vi "createDestinationDirectory.vi"(8 "error in (no error)":errorcluster, 11 "PolymorphicStructure in":refnum<class "PolymorphicStructure.lvclass">) -> (0 "error out":errorcluster, 2 "instanceDirectories":path[](array[path]), 3 "PolymorphicStructure out":refnum<class "PolymorphicStructure.lvclass">)   [LabVIEW 2012, in "PolymorphicStructure.lvclass"]
uses:
  PolymorphicStructure.lvclass
  PolymorphicStructure.lvclass/PolymorphicStructure.ctl
  <vilib>/LabVIEW Icon API/API_Text.ctl
  Directory/Directory.lvclass
  <vilib>/LabVIEW Icon API/LabVIEW Icon API.lvlib
  VirtualInstrument/VirtualInstrument.lvclass
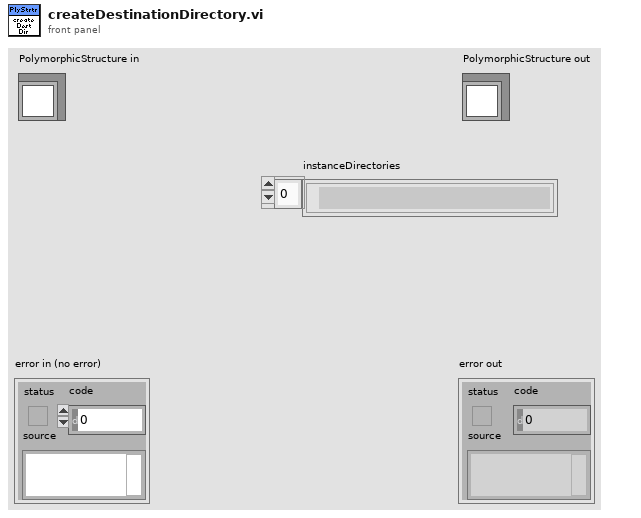
[diagram p1: front panel]
types:
  T1 = typedef "LabVIEW Icon API.lvlib/API_Text.ctl" = cluster{"Line 1 text":string, "Line 2 text":string, "Line 3 text":string, "Line 4 text":string}
  T2 = enum32{"invalid VI type", "Standard VI", "Control VI", "Global VI", "Polymorphic VI", "Configuration VI", "SubSystem", "Facade VI", "Method VI", "Statechart Diagram VI"}
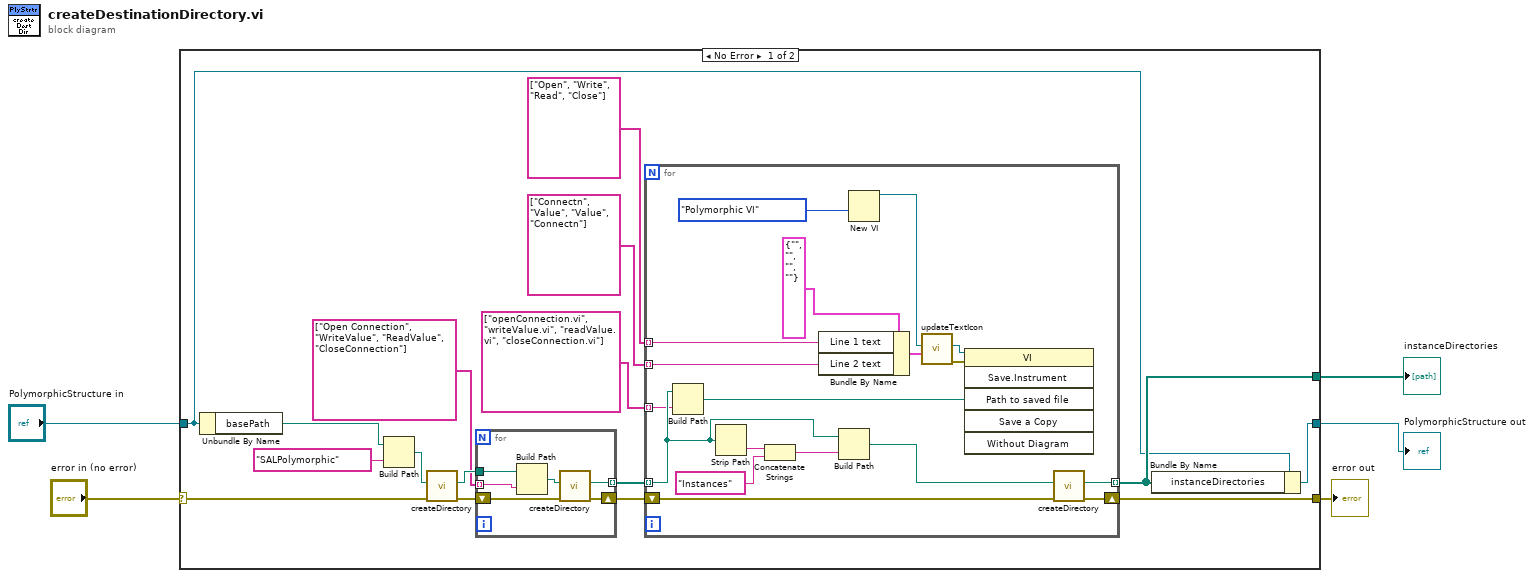
[diagram p0: block diagram]
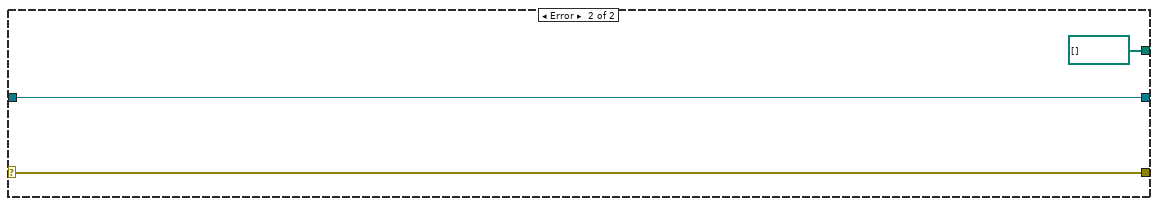
[diagram p2: hidden frame]
diagram:
  n1 = case shown="No Error" "error in (no error)" {
    selector: "error in (no error)" -> [w19 w48]
    tunnel: [w12 w48] -> w4
    tunnel: [w6 w47] -> w2
    tunnel: "PolymorphicStructure in" -> [w7 w47]
    tunnel: [w8 path[] []] -> w1
    frame No Error {
      n2 = Unbundle By Name(w7) -> ("basePath"=w21:path)
      n3 = Build Path(base path=w21, name or relative path="SALPolymorphic") -> (appended path=w18:path)
      n4 = call "createDirectory.vi"("error in (no error)"=w19, "newDirectoryPath"=w18) -> ("error out"=w15:errorcluster, "newDirectoryPath 2"=w17:path)  [unwired: 7 in, 1 out]
      n5 = for {
        tunnel: w17 -> [w45]
        tunnel: string[] ["Open Connection", "WriteValue", "ReadValue", "CloseConnection"] -> [w44] mode=indexing
        shift-right: [w41] -> w13
        shift-left: w15 -> [w42]
        tunnel: [w40] -> w14 mode=indexing
        n6 = Build Path(base path=w45, name or relative path=w44) -> (appended path=w43:path)
        n7 = call "createDirectory.vi"("error in (no error)"=w42, "newDirectoryPath"=w43) -> ("error out"=w41:errorcluster, "newDirectoryPath 2"=w40:path)  [unwired: 7 in, 1 out]
      }
      n8 = for {
        tunnel: w14 -> [w32] mode=indexing
        shift-right: [w34] -> w12
        shift-left: w13 -> [w35]
        tunnel: string[] ["openConnection.vi", "writeValue.vi", "readValue.vi", "closeConnection.vi"] -> [w30] mode=indexing
        tunnel: string[] ["Connectn", "Value", "Value", "Connectn"] -> [w29] mode=indexing
        tunnel: string[] ["Open", "Write", "Read", "Close"] -> [w28] mode=indexing
        tunnel: [w22] -> w8 mode=indexing
        n9 = Build Path(base path=w32, name or relative path=w30) -> (appended path=w31:path)
        n10 = Strip Path(path=w32) -> (name=w38:string)  [unwired: 1 out]
        n11 = Concatenate Strings(w38, "Instances" ("string")) -> (w36:string)
        n12 = Bundle By Name(cluster=T1 {"Line 1 text"="", "Line 2 text"="", "Line 3 text"="", "Line 4 text"=""} ("output cluster"), "Line 1 text"=w28, "Line 2 text"=w29) -> (w26:T1)
        n13 = Build Path(base path=w32, name or relative path=w36) -> (appended path=w39:path)
        n14 = New VI(9:T2."Polymorphic VI" ("vi type (standard vi)")) -> (3:w27:refnum<vi>)  [unwired: 6 in, 1 out]
        n15 = call "updateTextIcon.vi"("Text"=w26, "vi refnum"=w27) -> ("error out"=w24:errorcluster, "vi refnum 2"=w25:refnum<vi>)  [unwired: 7 in, 1 out]
        n16 = invoke class="VI" method="Save.Instrument"(reference=w25, error in=w24, "Path to saved file"=w31) -> ()  [unwired: 3 in, 6 out]
        n17 = call "createDirectory.vi"("error in (no error)"=w35, "newDirectoryPath"=w39) -> ("error out"=w34:errorcluster, "newDirectoryPath 2"=w22:path)  [unwired: 7 in, 1 out]
      }
      n18 = Bundle By Name(cluster=w7, "instanceDirectories"=w8) -> (w6:refnum<class "PolymorphicStructure.lvclass">)
    }
    frame Error {
    }
  }
  "error out" <- w4
  "PolymorphicStructure out" <- w2
  "instanceDirectories" <- w1
